vi "Address Page.vi"(8 "error in (no error)":errorcluster, 11 "Node Ptr":T1 format="%.0x") -> (0 "error out":errorcluster)   [LabVIEW 2013, in "J1939 Addon System Explorer.lvlib"]
uses:
  J1939 Addon System Explorer.lvlib
  <vilib>/NI Veristand/Custom Device API/Custom Device Item Ref.ctl
  Shared/Types/Monitor Settings.ctl
  Shared/SubVIs/Constants.vi
  <vilib>/NI Veristand/Custom Device API/Get Item Property (Variant).vi
  <vilib>/NI Veristand/Custom Device API/Set Item Property (Variant).vi
  <vilib>/NI Veristand/Custom Device API/Custom Device API.lvlib
  Shared/J1939 Addon Shared.lvlib
panel:
  in  "Settings":cluster{"Section Name":string}={"Section Name"="Address Settings"}
  in  "J1939 Name":u64 format="%.0x"
  in  "J1939 Network Address":u8
  in  "Description":string
  in  "Name":string
  in  "SHDocVw.IWebBrowser2":refnum<k7>(container)
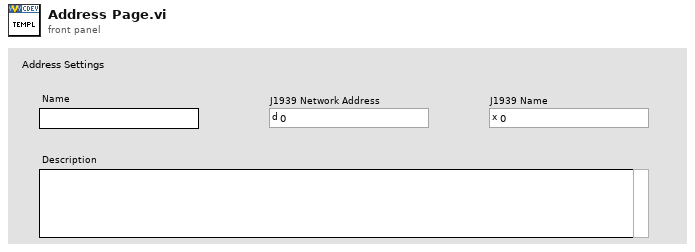
[diagram p1: front panel]
types:
  T1 = typedef "Custom Device API.lvlib/Custom Device Item Ref.ctl" = u64
  T2 = typedef "J1939 Addon Shared.lvlib/Monitor Settings.ctl" = cluster{"J1939 Network Address":u8, "Name":u64}
  T3 = typedef "Custom Device API.lvlib/Custom Device Item Info.ctl" = cluster{"Name":string, "Is Channel":bool, "GUID":string, "Is Waveform":bool}
  T4 = typedef "Custom Device API.lvlib/Custom Device Commands.ctl" = enum16{"Default", "Item renamed", "Shutdown", "Dynamic button pressed"}
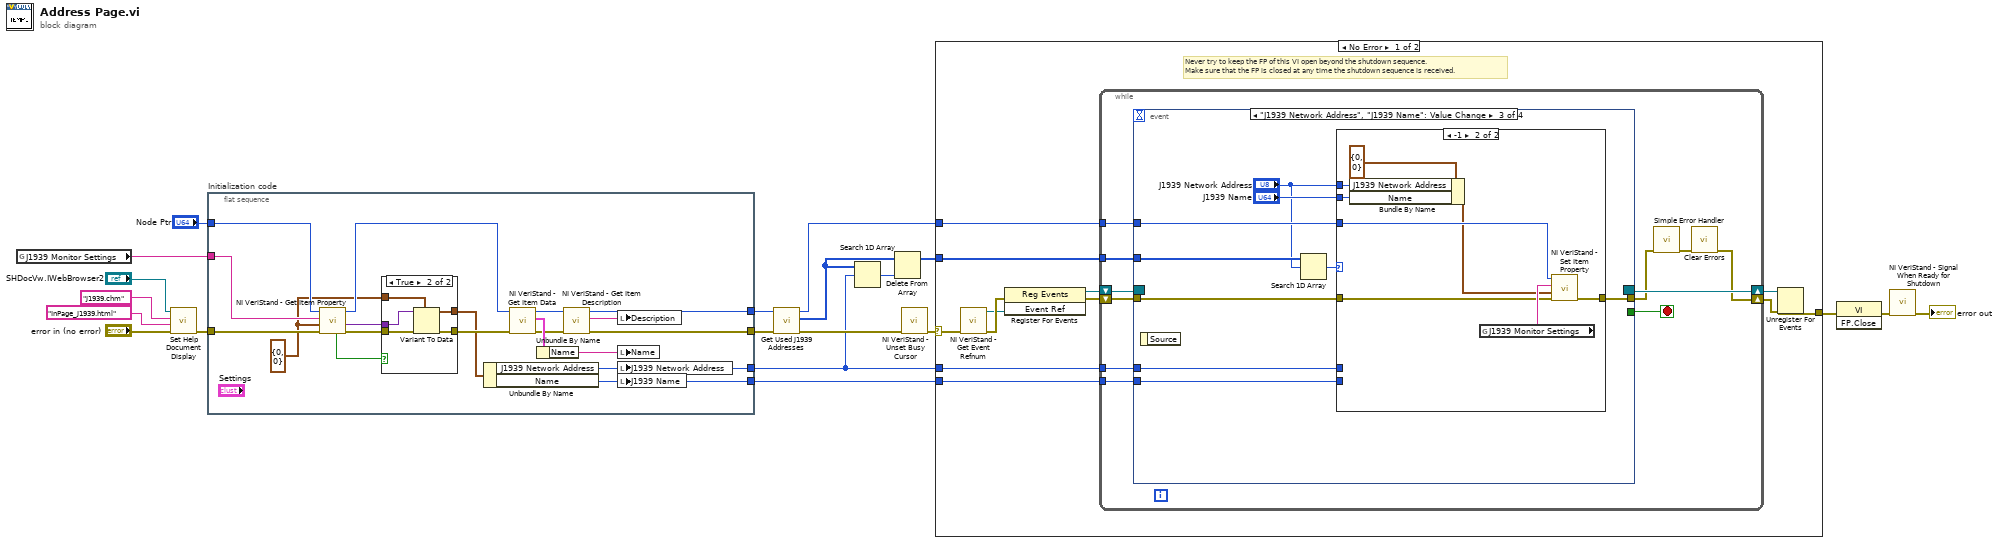
[diagram p0: block diagram]
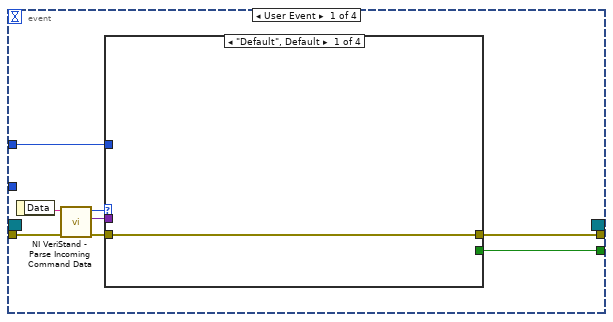
[diagram p2: hidden frame]
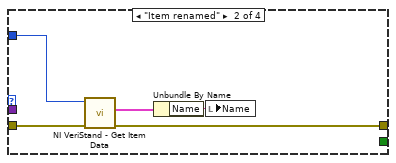
[diagram p3: hidden frame]
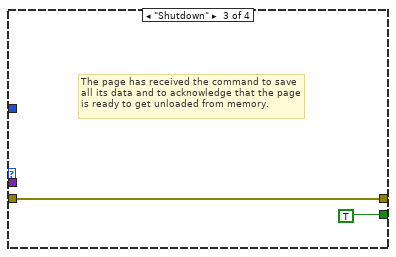
[diagram p4: hidden frame]
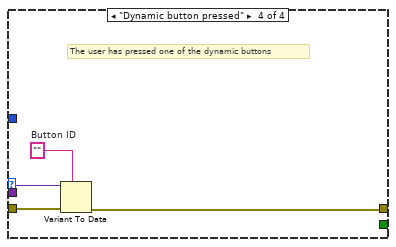
[diagram p5: hidden frame]
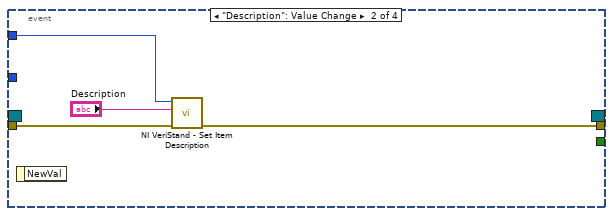
[diagram p6: hidden frame]
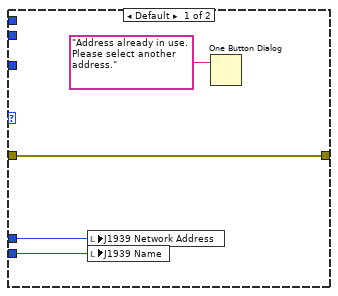
[diagram p7: hidden frame]
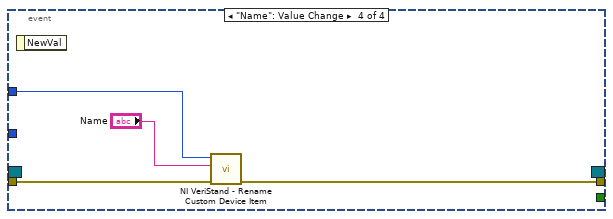
[diagram p8: hidden frame]
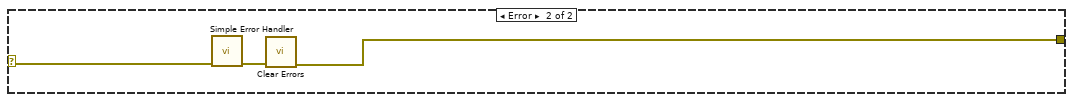
[diagram p9: hidden frame]
diagram:
  n1 = global read "Constants.vi" "J1939 Monitor Settings"() -> (w10:string)
  n2 = call "Set Help Document Display.vi"("error in (no error)"="error in (no error)", "HTML File"="InPage_J1939.html", "Main CHM File"="J1939.chm", "SHDocVw.IWebBrowser2"="SHDocVw.IWebBrowser2") -> ("error out"=w11:errorcluster)  [unwired: 7 in]
  n3 = flat-sequence "Initialization code" {
    tunnel: w11 -> [w32]
    tunnel: "Node Ptr" -> [w30]
    tunnel: [w36] -> w8
    tunnel: [w34] -> w6
    tunnel: w10 -> [w28]
    tunnel: [w22] -> w2
    tunnel: [w21] -> w1
    frame #0 {
      w24 = T2 {"J1939 Network Address"=0, "Name"=0} ("J1939 XNET Settings")
      n4 = call-poly <vilib>:"NI VeriStand - Get Item Property.vi"("error in (no error)"=w32, "Default Value"=w24, "Property Name"=w28, "Item Ref in"=w30) -> ("error out"=w31:errorcluster, "Value"=w26:variant, "Item Ref out"=w29:T1, "Found?"=w25:bool)  [unwired: 4 in]
      n5 = case shown="True" w25 {
        tunnel: w31 -> [w41 w46]
        tunnel: [w41 w45] -> w27
        tunnel: w26 -> [_ w44]
        tunnel: w24 -> [w40 w43]
        tunnel: [w40 w42] -> w23
        frame False {
        }
        frame True {
          n6 = Variant To Data(error in=w46, type=w43, Variant=w44) -> (data=w42:T2, error out=w45:errorcluster)
        }
      }
      n7 = Unbundle By Name(w23) -> ("J1939 Network Address"=w22:u8, "Name"=w21:u64)
      n8 = call <vilib>:"NI VeriStand - Get Item Data.vi"("error in (no error)"=w27, "Item Ref in"=w29) -> ("error out"=w37:errorcluster, "Item Info"=w39:T3, "Item Ref out"=w35:T1)  [unwired: 7 out]
      n9 = Unbundle By Name(w39) -> ("Name"=w38:string)
      n10 = call <vilib>:"NI VeriStand - Get Item Description.vi"("error in (no error)"=w37, "Item Ref in"=w35) -> ("error out"=w36:errorcluster, "Description"=w33:string, "Item Ref out"=w34:T1)  [unwired: 6 in, 1 out]
      n11 = local write "Description"(w33) -> ()
      n12 = local write "Name"(w38) -> ()
      n13 = local write "J1939 Network Address"(w22) -> ()
      n14 = local write "J1939 Name"(w21) -> ()
    }
  }
  n15 = call "Get Used J1939 Addresses.vi"("error in (no error)"=w8, "Node Ptr"=w6) -> ("error out"=w9:errorcluster, "Addresses"=w5:u8[], "Item Ref out"=w7:T1)  [unwired: 7 in]
  n16 = Search 1D Array(1D array=w5, element=w2) -> (index of element=w4:i32)  [unwired: 1 in]
  n17 = Delete From Array(array=w5, index=w4) -> (array with subset deleted=w3:u8[])  [unwired: 1 in, 1 out]
  n18 = call <vilib>:"NI VeriStand - Unset Busy Cursor.vi"("error in (no error)"=w9) -> ("error out"=w16:errorcluster)  [unwired: 10 out]
  n19 = case shown="No Error" w16 {
    selector: w16 -> [w50 w121]
    tunnel: [w55 w119] -> w20
    tunnel: w7 -> [w51 _]
    tunnel: w3 -> [w49 _]
    tunnel: w2 -> [w48 _]
    tunnel: w1 -> [w47 _]
    frame No Error {
      # "Never try to keep the FP of this VI open beyond the shutdown sequence.\nMake sure that the FP is closed at any time the shutdown sequence is received."
      n20 = call <vilib>:"NI VeriStand - Get Event Refnum.vi"("error in (no error)"=w50) -> ("error out"=w58:errorcluster, "Event Ref"=w54:refnum<user-event>)  [unwired: 9 out]
      n21 = register-events(error in=w58, w54) -> (reference out=w52:refnum<event-registration>, error out=w53:errorcluster)  [unwired: 1 in]
      n22 = while {
        tunnel: w51 -> [w65]
        shift-right: [w62] -> w56
        shift-left: w53 -> [w68]
        shift-right: [w69] -> w57
        shift-left: w52 -> [w67]
        tunnel: w49 -> [w61]
        tunnel: w48 -> [w60]
        tunnel: w47 -> [w59]
        stop <- w66 stop-if-true
        n23 = event shown="[2] \"J1939 Network Address\", \"J1939 Name\": Value Change" {
          selector: w67 -> [_ _ _ _]
          dyn-events: [_ _ _ _] -> w69
          timeout: _ -> [_ _ _ _]
          tunnel: w68 -> [w77 w93 w101 w118]
          tunnel: [w73 _ _ _] -> w66
          tunnel: [w72 w90 w100 w116] -> w64
          tunnel: w65 -> [w71 w91 w99 w117]
          tunnel: w61 -> [_ _ w98 _]
          tunnel: w60 -> [_ _ w95 _]
          tunnel: w59 -> [_ _ w94 _]
          event User Event {
            n24 = event-data() -> ("Data"=w76:string)  [unwired: 1 out]
            n25 = call <vilib>:"NI VeriStand - Parse Incoming Command Data.vi"("error in (no error)"=w77, "Incoming data"=w76) -> ("error out"=w75:errorcluster, "Outgoing data"=w70:variant, "Action"=w74:T4)  [unwired: 7 out]
            n26 = case shown="\"Default\", Default" w74 {
              tunnel: w75 -> [w78 w81 w84 w89]
              tunnel: [_ _ TRUE _] -> w73
              tunnel: [w78 w79 w84 w86] -> w72
              tunnel: w71 -> [_ w80 _ _]
              tunnel: w70 -> [_ _ _ w88]
              frame "Default", Default {
              }
              frame "Item renamed" {
                n27 = call <vilib>:"NI VeriStand - Get Item Data.vi"("error in (no error)"=w81, "Item Ref in"=w80) -> ("error out"=w79:errorcluster, "Item Info"=w82:T3)  [unwired: 8 out]
                n28 = Unbundle By Name(w82) -> ("Name"=w83:string)
                n29 = local write "Name"(w83) -> ()
              }
              frame "Shutdown" {
                # "The page has received the command to save all its data and to acknowledge that the page is ready to get unloaded from memory."
              }
              frame "Dynamic button pressed" {
                w87 = ""  # Button ID
                # "The user has pressed one of the dynamic buttons"
                n30 = Variant To Data(error in=w89, type=w87, Variant=w88) -> (error out=w86:errorcluster)  [unwired: 1 out]
              }
            }
          }
          event "Description": Value Change {
            n31 = event-data() -> ()  [unwired: 2 out]
            n32 = call <vilib>:"NI VeriStand - Set Item Description.vi"("error in (no error)"=w93, "Description"="Description", "Item Ref in"=w91) -> ("error out"=w90:errorcluster)  [unwired: 6 in, 2 out]
          }
          event "J1939 Network Address", "J1939 Name": Value Change {
            n33 = event-data() -> ()  [unwired: 2 out]
            n34 = Search 1D Array(1D array=w98, element="J1939 Network Address") -> (index of element=w96:i32)  [unwired: 1 in]
            n35 = case shown="-1" w96 {
              tunnel: "J1939 Name" -> [_ w114]
              tunnel: w101 -> [w106 w111]
              tunnel: [w106 w110] -> w100
              tunnel: w99 -> [_ w109]
              tunnel: "J1939 Network Address" -> [_ w107]
              tunnel: w95 -> [w104 _]
              tunnel: w94 -> [w103 _]
              frame Default {
                n36 = local write "J1939 Network Address"(w104) -> ()
                n37 = local write "J1939 Name"(w103) -> ()
                n38 = One Button Dialog(message="Address already in use. Please select another address.") -> ()  [unwired: 1 in, 1 out]
              }
              frame -1 {
                n39 = Bundle By Name(cluster=T2 {"J1939 Network Address"=0, "Name"=0} ("J1939 XNET Settings"), "J1939 Network Address"=w107, "Name"=w114) -> (w108:T2)
                n40 = global read "Constants.vi" "J1939 Monitor Settings"() -> (w112:string)
                n41 = call-poly <vilib>:"NI VeriStand - Set Item Property.vi"("error in (no error)"=w111, "Value"=w108, "Property Name"=w112, "Item Ref in"=w109) -> ("error out"=w110:errorcluster)  [unwired: 5 in, 2 out]
              }
            }
          }
          event "Name": Value Change {
            n42 = event-data() -> ()  [unwired: 2 out]
            n43 = call <vilib>:"NI VeriStand - Rename Custom Device Item.vi"("error in (no error)"=w118, "New Name"="Name", "Item Ref in"=w117) -> ("error out"=w116:errorcluster)  [unwired: 1 in, 7 out]
          }
        }
        n44 = call <vilib>:"Simple Error Handler.vi"("error in (no error)"=w64) -> ("error out"=w63:errorcluster)  [unwired: 1 in, 7 out]
        n45 = call <vilib>:"Clear Errors.vi"("error in (no error)"=w63) -> ("error out"=w62:errorcluster)  [unwired: 6 out]
      }
      n46 = Unregister For Events(event registration refnum=w57, error in=w56) -> (error out=w55:errorcluster)
    }
    frame Error {
      n47 = call <vilib>:"Simple Error Handler.vi"("error in (no error)"=w121) -> ("error out"=w120:errorcluster)  [unwired: 1 in, 7 out]
      n48 = call <vilib>:"Clear Errors.vi"("error in (no error)"=w120) -> ("error out"=w119:errorcluster)  [unwired: 6 out]
    }
  }
  n49 = invoke class="VI" method="FP.Close"(error in=w20) -> (error out=w19:errorcluster)  [unwired: 2 in, 2 out]
  n50 = call <vilib>:"NI VeriStand - Signal When Ready for Shutdown.vi"("error in (no error)"=w19) -> ("error out"=→"error out":errorcluster)  [unwired: 10 out]
